vi "Vision Research Phantom Series PhCon PhRecordSpecificCine.vi"(0 "CN in":u32=1, 2 "Cine":i32, 5 "Error In (no error)":errorcluster) -> (14 "CN out":u32=1, 19 "Error Out":errorcluster)   [LabVIEW 2013, in "VRI.lvlib"]
doc: "PhCon.dll\n\nPhRecordSpecificCine\nHRESULT PhRecordSpecificCine(UINT CN, int Cine)\n\nParameters Description\nCN (in) Camera number.\nCine (in) Cine number where to start the recording.\nReturn HRESULT (0 = Ok)\nComments Starts a recording in a specified partition of a multicine\n camera. Deletes the existing cine if there is one\n recorded."
uses:
  VRI.lvlib
  Phantom DLLs/PhCon.Dll
panel:
  # "For instructions on the use of this VI, press Ctrl+H to display the help window and move the mouse over the icon, controls, and indicators"
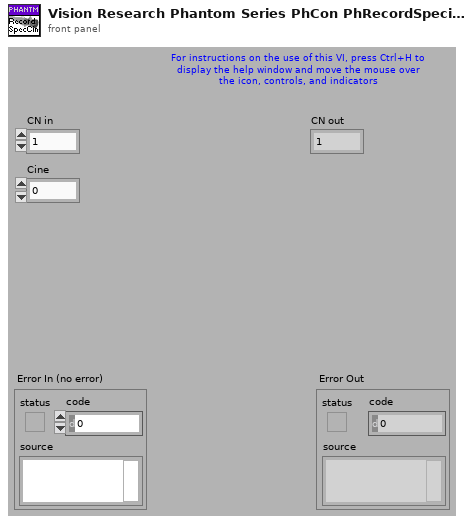
[diagram p1: front panel]
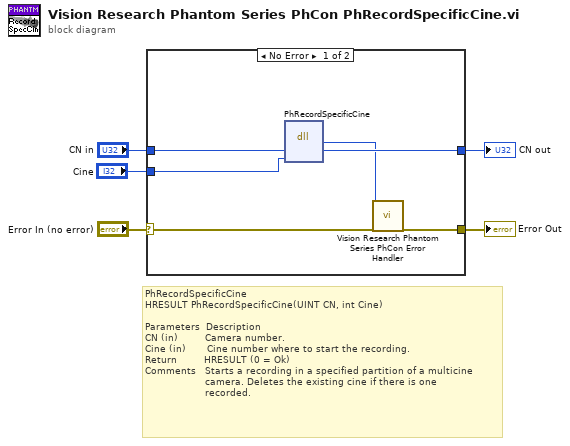
[diagram p0: block diagram]
diagram:
  # "PhRecordSpecificCine\nHRESULT PhRecordSpecificCine(UINT CN, int Cine)\n\nParameters  Description\nCN (in)         Camera number.\nCine (in)       Cine number where to start the recording.\nReturn         HRESULT (0 = Ok)\nComments   Starts a recording in a specified partition of a multicine\n                    camera. Deletes the existing cine if there is one\n                    recorded."
  n1 = case shown="No Error" "Error In (no error)" {
    selector: "Error In (no error)" -> [w11 w13]
    tunnel: [w10 w13] -> w4
    tunnel: "CN in" -> [w9 w12]
    tunnel: [w8 w12] -> w2
    tunnel: "Cine" -> [w7 _]
    frame No Error {
      n2 = dll-call lib="C:/Projects/SDK/64-bit/Vision Research Phantom Series Labview Driver/Phantom DLLs/PhCon.dll" fn="PhRecordSpecificCine"("CN"=w9, "Cine"=w7) -> ("HRESULT"=w6:i32, "CN"=w8:u32)  [unwired: 4 in, 2 out]
      n3 = call "Vision Research Phantom Series PhCon Error Handler.vi"("ErrNo"=w6, "Error In (no error)"=w11) -> ("Error Out"=w10:errorcluster)  [unwired: 17 out]
    }
    frame Error {
    }
  }
  "Error Out" <- w4
  "CN out" <- w2
